vi "MultiTableGenerateNameAndHeaders.vi"(8 "error in (no error)":errorcluster, 9 "Array Call":bool, 10 "Incl. Top-Level Table Name":bool=TRUE, 11 "Cluster Variant":variant) -> (0 "error out":errorcluster, 1 "SQL Data Types":string[][](array[string]), 2 "Headers":string[][](array[string]), 3 "Table Names":string[](array[string]), 5 "LV Data Types":T1[][](array[typedef]) format="%.0x")   [LabVIEW 2014, in "TableLogger_Actor.lvlib" / "TableLogger_Actor.lvclass"]
uses:
  TableLogger_Actor.lvclass
  <userlib>/_OpenG.lib/lvdata/lvdata.llb/Type Descriptor Enumeration__ogtk.ctl
panel:
  # "Connector Pane"
  # "Locals"
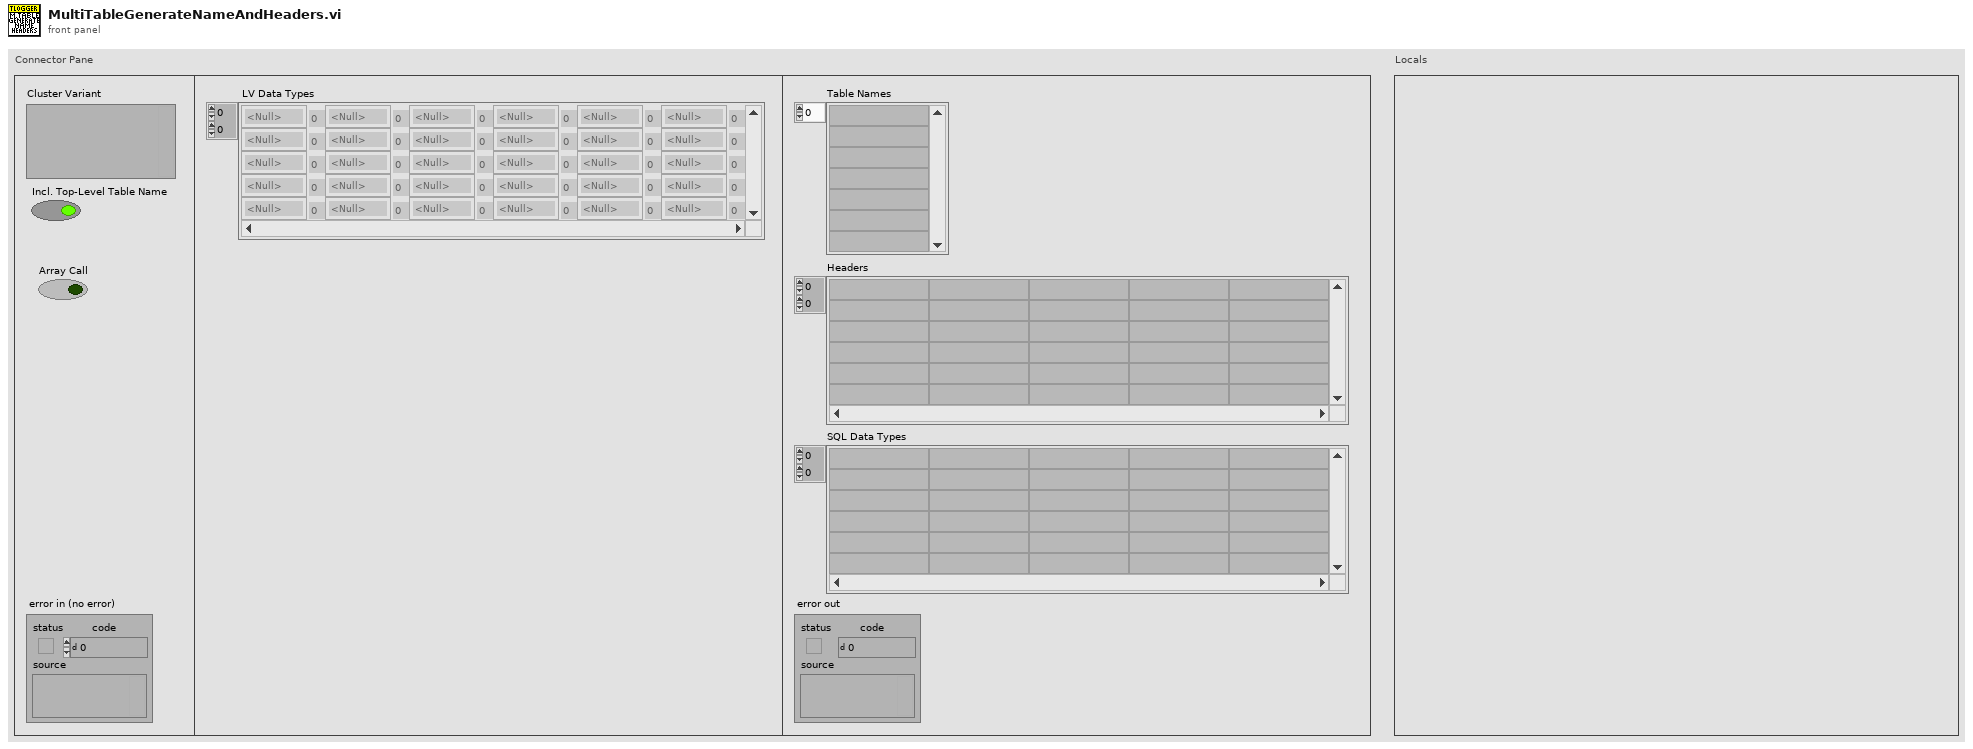
[diagram p1: front panel]
types:
  T1 = typedef "Type Descriptor Enumeration__ogtk.ctl" = enum8{"<Null>", "I8", "I16", "I32", "I64", "U8", "U16", "U32", "U64", "SGL", "DBL", "EXT", "CSG", "CDB", "CXT", "0x0F", "0x10", "0x11", "0x12", "0x13", "0x14", "Enum U8", "Enum U16", "Enum U32", "Enum U64", "SGL PQ", "DBL PQ", "EXT PQ", "CSG PQ", "CDB PQ", "CXT PQ", "0x1F", "0x20", "Boolean", "0x22", "0x23", "0x24", "0x25", "0x26", "0x27", "0x28", "0x29", "0x2A", "0x2B", "0x2C", "0x2D", "0x2E", "0x2F", "String", "0x31", "Path", "Pict", "0x34", "0x35", "0x36", "DAQ", "0x38", "0x39", "0x3A", "0x3B", "0x3C", "0x3D", "0x3E", "0x3F", "Array", "0x41", "0x42", "0x43", "0x44", "0x45", "0x46", "0x47", "0x48", "0x49", "0x4A", "0x4B", "0x4C", "0x4D", "0x4E", "0x4F", "Cluster", "0x51", "0x52", "Variant", "Waveform", "0x55", "0x56", "0x57", "0x58", "0x59", "0x5A", "0x5B", "0x5C", "0x5D", "0x5E", "0x5F", "0x60", "0x61", "0x62", "0x63", "0x64", "0x65", "0x66", "0x67", "0x68", "0x69", "0x6A", "0x6B", "0x6C", "0x6D", "0x6E", "0x6F", "Refnum"}
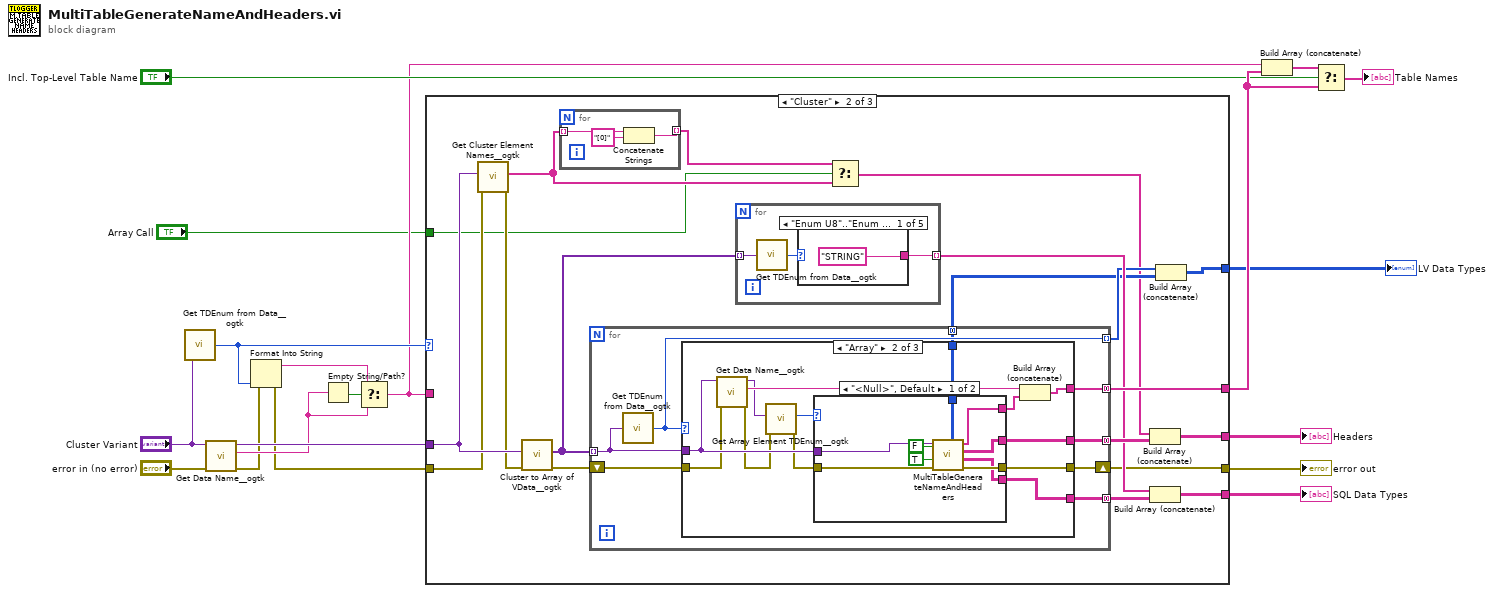
[diagram p0: block diagram]
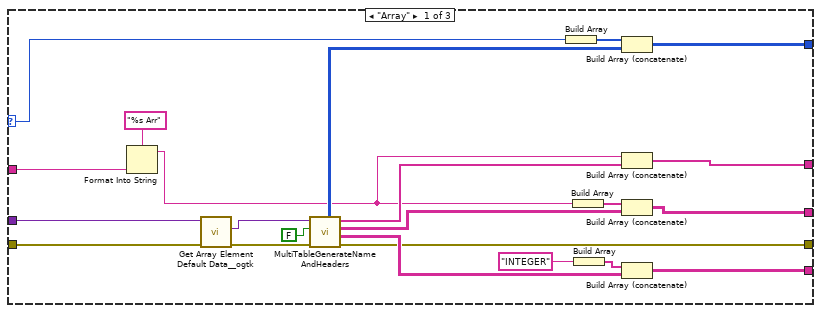
[diagram p2: hidden frame]
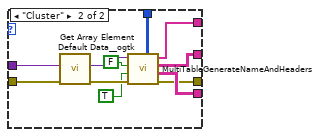
[diagram p4: hidden frame]
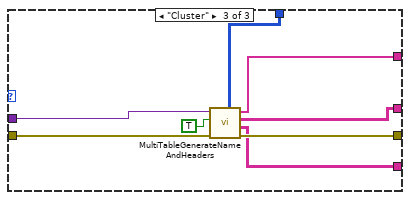
[diagram p5: hidden frame]
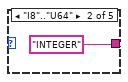
[diagram p6: hidden frame]
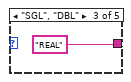
[diagram p7: hidden frame]
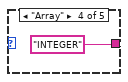
[diagram p8: hidden frame]
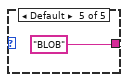
[diagram p9: hidden frame]
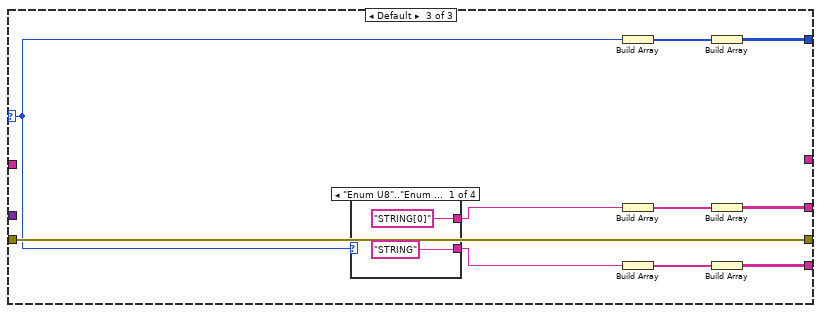
[diagram p10: hidden frame]
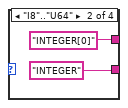
[diagram p11: hidden frame]
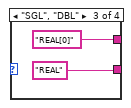
[diagram p12: hidden frame]
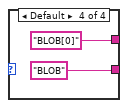
[diagram p13: hidden frame]
diagram:
  n1 = call <userlib>:"Get TDEnum from Data__ogtk.vi"("Data"="Cluster Variant") -> ("Type Descriptor Enumeration"=w6:T1)  [unwired: 4 in]
  n2 = call <userlib>:"Get Data Name__ogtk.vi"("error in (no error)"="error in (no error)", "Data"="Cluster Variant") -> ("error out"=w4:errorcluster, "Data Name"=w7:string, "Data dup"=w9:variant)  [unwired: 7 in]
  n3 = Format Into String(error in=w4, w6) -> (resulting string=w5:string, error out=w3:errorcluster)  [unwired: 2 in]
  n4 = Empty String/Path?(string/path=w7) -> (empty?=w8:bool)
  n5 = Select(t=w5, s=w8, f=w7) -> (s? t:f=w2:string)
  n6 = case shown="\"Cluster\"" w6 {
    selector: w6 -> [w28 _ w123]
    tunnel: w9 -> [w25 w57 _]
    tunnel: [w36 w56 w126] -> w19
    tunnel: [w34 w55 w125] -> w18
    tunnel: [w22 w58 _] -> w14
    tunnel: w3 -> [w26 w51 w131]
    tunnel: [w37 w49 w131] -> w17
    tunnel: [w30 w47 w122] -> w12
    tunnel: w2 -> [w20 _ _]
    tunnel: "Array Call" -> [_ w42 _]
    frame "Array" {
      n7 = Format Into String(format string="%s Arr", w20) -> (resulting string=w21:string)  [unwired: 2 in, 1 out]
      n8 = call <userlib>:"Get Array Element Default Data__ogtk.vi"("error in (no error)"=w26, "Array"=w25) -> ("error out"=w24:errorcluster, "Array Element Default Data"=w27:variant)  [unwired: 8 in]
      n9 = call "MultiTableGenerateNameAndHeaders.vi"("error in (no error)"=w24, "Incl. Top-Level Table Name"=FALSE, "Cluster Variant"=w27) -> ("error out"=w37:errorcluster, "SQL Data Types"=w38:string[][], "Headers"=w39:string[][], "Table Names"=w40:string[], "LV Data Types"=w31:T1[][])  [unwired: 4 in]
      n10 = Build Array(w28) -> (w29:T1[])
      n11 = Build Array(w21) -> (w35:string[])
      n12 = Build Array("INTEGER") -> (w33:string[])
      n13 = Build Array (concatenate)(w29, w31) -> (w30:T1[][])
      n14 = Build Array (concatenate)(w21, w40) -> (w22:string[])
      n15 = Build Array (concatenate)(w35, w39) -> (w36:string[][])
      n16 = Build Array (concatenate)(w33, w38) -> (w34:string[][])
    }
    frame "Cluster" {
      n17 = call <userlib>:"Get Cluster Element Names__ogtk.vi"("error in (no error)"=w51, "Cluster"=w57) -> ("error out"=w52:errorcluster, "Element Names"=w43:string[])  [unwired: 8 in]
      n18 = call <userlib>:"Cluster to Array of VData__ogtk.vi"("error in (no error)"=w52, "Cluster"=w57) -> ("error out"=w50:errorcluster, "Array of VData"=w54:variant[])  [unwired: 8 in]
      n19 = for {
        tunnel: w43 -> [w63] mode=indexing
        tunnel: [w62] -> w44 mode=indexing
        n20 = Concatenate Strings(w63, "[0]" ("string")) -> (w62:string)
      }
      n21 = for {
        tunnel: w54 -> [w71] mode=indexing
        tunnel: [w70] -> w60 mode=concatenating
        tunnel: [w69] -> w58 mode=concatenating
        tunnel: [w68] -> w59 mode=concatenating
        shift-right: [w66] -> w49
        shift-left: w50 -> [w67]
        tunnel: [w65] -> w48 mode=indexing
        tunnel: [w64] -> w46 mode=concatenating
        n22 = call <userlib>:"Get TDEnum from Data__ogtk.vi"("Data"=w71) -> ("Type Descriptor Enumeration"=w65:T1)  [unwired: 4 in]
        n23 = case shown="\"Array\"" w65 {
          tunnel: w71 -> [_ w83 w113]
          tunnel: [_ w84 w108] -> w70
          tunnel: [_ w81 w109] -> w69
          tunnel: [_ w79 w107] -> w68
          tunnel: w67 -> [w72 w77 w111]
          tunnel: [w72 w74 w110] -> w66
          tunnel: [_ w73 w106] -> w64
          frame Default {
          }
          frame "Array" {
            n24 = call <userlib>:"Get Data Name__ogtk.vi"("error in (no error)"=w77, "Data"=w83) -> ("error out"=w78:errorcluster, "Data Name"=w82:string, "Data dup"=w76:variant)  [unwired: 7 in]
            n25 = call <userlib>:"Get Array Element TDEnum__ogtk.vi"("error in (no error)"=w78, "Array"=w76) -> ("error out"=w75:errorcluster, "Element Type"=w85:T1)  [unwired: 8 in]
            n26 = case shown="\"<Null>\", Default" w85 {
              tunnel: w83 -> [w88 w105]
              tunnel: [w90 w100] -> w84
              tunnel: [w91 w101] -> w80
              tunnel: [w89 w102] -> w79
              tunnel: w75 -> [w94 w99]
              tunnel: [w93 w97] -> w74
              tunnel: [w92 w96] -> w73
              frame "<Null>", Default {
                n27 = call "MultiTableGenerateNameAndHeaders.vi"("error in (no error)"=w94, "Array Call"=TRUE, "Incl. Top-Level Table Name"=FALSE, "Cluster Variant"=w88) -> ("error out"=w93:errorcluster, "SQL Data Types"=w89:string[][], "Headers"=w90:string[][], "Table Names"=w91:string[], "LV Data Types"=w92:T1[][])  [unwired: 3 in]
              }
              frame "Cluster" {
                n28 = call <userlib>:"Get Array Element Default Data__ogtk.vi"("error in (no error)"=w99, "Array"=w105) -> ("error out"=w98:errorcluster, "Array Element Default Data"=w104:variant)  [unwired: 8 in]
                n29 = call "MultiTableGenerateNameAndHeaders.vi"("error in (no error)"=w98, "Array Call"=TRUE, "Incl. Top-Level Table Name"=FALSE, "Cluster Variant"=w104) -> ("error out"=w97:errorcluster, "SQL Data Types"=w102:string[][], "Headers"=w100:string[][], "Table Names"=w101:string[], "LV Data Types"=w96:T1[][])  [unwired: 3 in]
              }
            }
            n30 = Build Array (concatenate)(w82, w80) -> (w81:string[])
          }
          frame "Cluster" {
            n31 = call "MultiTableGenerateNameAndHeaders.vi"("error in (no error)"=w111, "Incl. Top-Level Table Name"=TRUE, "Cluster Variant"=w113) -> ("error out"=w110:errorcluster, "SQL Data Types"=w107:string[][], "Headers"=w108:string[][], "Table Names"=w109:string[], "LV Data Types"=w106:T1[][])  [unwired: 4 in]
          }
        }
      }
      n32 = for {
        tunnel: w54 -> [w116] mode=indexing
        tunnel: [w114] -> w53 mode=indexing
        n33 = call <userlib>:"Get TDEnum from Data__ogtk.vi"("Data"=w116) -> ("Type Descriptor Enumeration"=w115:T1)  [unwired: 4 in]
        n34 = case shown="\"Enum U8\"..\"Enum U64\", \"String\", \"Waveform\"" w115 {
          tunnel: ["STRING" "INTEGER" "REAL" "INTEGER" "BLOB"] -> w114
          frame "Enum U8".."Enum U64", "String", "Waveform" {
          }
          frame "I8".."U64" {
          }
          frame "SGL", "DBL" {
          }
          frame "Array" {
          }
          frame Default {
          }
        }
      }
      n35 = Select(t=w44, s=w42, f=w43) -> (s? t:f=w45:string[])
      n36 = Build Array (concatenate)(w45, w60) -> (w56:string[][])
      n37 = Build Array (concatenate)(w53, w59) -> (w55:string[][])
      n38 = Build Array (concatenate)(w48, w46) -> (w47:T1[][])
    }
    frame Default {
      n39 = case shown="\"Enum U8\"..\"Enum U64\", \"String\", \"Waveform\"" w123 {
        tunnel: ["STRING" "INTEGER" "REAL" "BLOB"] -> w129
        tunnel: ["STRING[0]" "INTEGER[0]" "REAL[0]" "BLOB[0]"] -> w130
        frame "Enum U8".."Enum U64", "String", "Waveform" {
        }
        frame "I8".."U64" {
        }
        frame "SGL", "DBL" {
        }
        frame Default {
        }
      }
      n40 = Build Array(w123) -> (w124:T1[])
      n41 = Build Array(w130) -> (w127:string[])
      n42 = Build Array(w129) -> (w128:string[])
      n43 = Build Array(w124) -> (w122:T1[][])
      n44 = Build Array(w127) -> (w126:string[][])
      n45 = Build Array(w128) -> (w125:string[][])
    }
  }
  "Headers" <- w19
  "SQL Data Types" <- w18
  "error out" <- w17
  "LV Data Types" <- w12
  n46 = Build Array (concatenate)(w2, w14) -> (w15:string[])
  n47 = Select(t=w15, s="Incl. Top-Level Table Name", f=w14) -> (s? t:f=→"Table Names":string[])
